vi "cos_rise.vi"(9 "new step":bool, 10 "change rate":u16, 11 "data in":fxp<+/-,16,1>) -> (2 "steping":bool, 3 "data out":fxp<+/-,16,1>)   [LabVIEW 2021]
doc: "rise function.\n32 steps of half cos."
uses:
  <instrlib>/_niInstr/Basic Elements/v1/FPGA/Private/Count Up U8.vi
  <instrlib>/_niInstr/Basic Elements/v1/FPGA/Private/Count Up U16.vi
  <vilib>/rvi/FXPMathLib/FxpSub/XNode/nifxpmath_Sub.xnode
  <vilib>/rvi/FXPMathLib/FxpMul/XNode/nifxpmath_Multiplier.xnode
  <vilib>/rvi/FXPMathLib/FxpAdd/XNode/nifxpmath_Add.xnode
  <instrlib>/_niInstr/Basic Elements/v1/FPGA/niInstr Basic Elements v1 FPGA.lvlib
  <vilib>/rvi/FXPMathLib/sim/FxpSim.dll
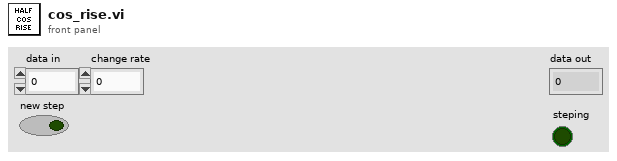
[diagram p1: front panel]
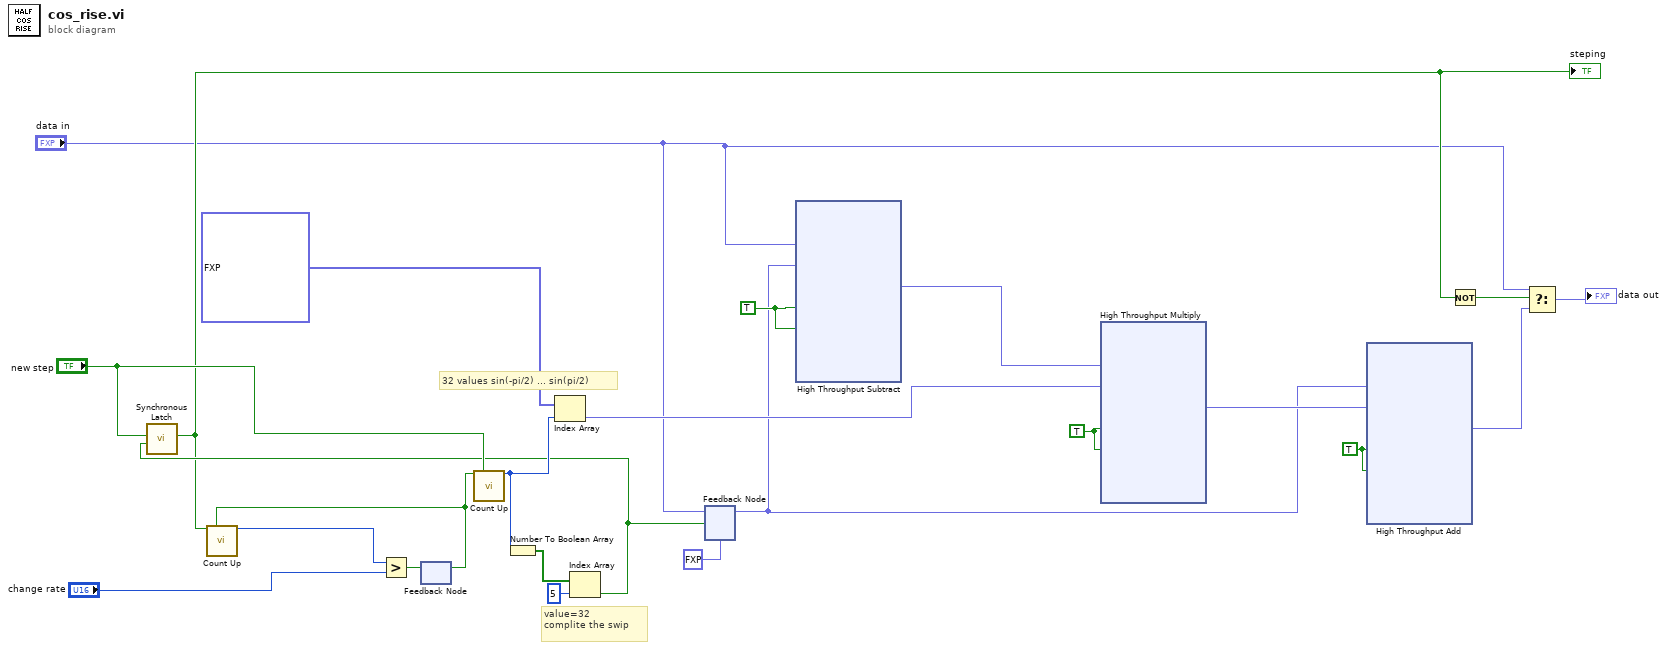
[diagram p0: block diagram]
diagram:
  w5 = TRUE ("input valid")
  w19 = TRUE ("input valid")
  w22 = TRUE ("input valid")
  # "value=32\ncomplite the swip"
  # "32 values sin(-pi/2) ... sin(pi/2)"
  n1 = feedback #1() -> (w15:bool)  [unwired: 1 in]
  n2 = call-poly <instrlib>:"Count Up.vi"("increment"=w15, "reset"="new step") -> ("count out"=w11:u8)  [unwired: 13 in]
  n3 = Number To Boolean Array(number=w11) -> (Boolean array=w10:bool[])
  n4 = Index Array(array=fxp<+/-,32,16>[] [0.0, 0.0025634765625, 0.0102386474609375, 0.0229339599609375, 0.04052734375, 0.0628204345703125, 0.0896148681640625, 0.1206207275390625, 0.155517578125, 0.1939544677734375, 0.2355194091796875, 0.2798004150390625, 0.32635498046875, 0.3746795654296875, 0.424285888671875, 0.47467041015625, 0.52532958984375, 0.575714111328125, 0.6253204345703125, 0.67364501953125, 0.7201995849609375, 0.7644805908203125, 0.8060455322265625, 0.844482421875, 0.8793792724609375, 0.9103851318359375, 0.9371795654296875, 0.95947265625, 0.9770660400390625, 0.9897613525390625, 0.9974365234375, 0.9999847412109375] ("Array 2"), index=w11) -> (element=w23:fxp<+/-,32,16>)
  n5 = Index Array(array=w10, index=5) -> (element=w8:bool)
  n6 = call <instrlib>:"Synchronous Latch.vi"("clear"=w8, "set"="new step") -> ("out"=w6:bool)  [unwired: 9 in]
  "steping" <- w6
  n7 = call-poly <instrlib>:"Count Up.vi"("increment"=w6, "reset"=w15) -> ("count out"=w18:u16)  [unwired: 13 in]
  n8 = Greater?(x=w18, y="change rate") -> (0:w16:bool)
  n9 = feedback-in #1(w16) -> ()
  n10 = feedback-in #2("data in", w8) -> ()
  n11 = feedback #2(fxp<+/-,16,1> 0.0 ("data in")) -> (w2:fxp<+/-,16,1>)
  n12 = xnode "High Throughput Subtract"("x"="data in", "y"=w2, "input valid"=w19, "ready for output (T)"=w19) -> ("x-y"=w20:fxp<+/-,16,1>)  [unwired: 2 out]
  n13 = xnode "High Throughput Multiply"("x"=w20, "y"=w23, "input valid"=w22, "ready for output (T)"=w22) -> ("x*y"=w21:fxp<+/-,16,1>)  [unwired: 2 out]
  n14 = xnode "High Throughput Add"("x"=w2, "y"=w21, "input valid"=w5, "ready for output (T)"=w5) -> ("x+y"=w14:fxp<+/-,16,1>)  [unwired: 2 out]
  n15 = Not(x=w6) -> (.not. x?=w7:bool)
  n16 = Select(t="data in", s=w7, f=w14) -> (s? t:f=→"data out":fxp<+/-,16,1>)
